vi "Set Cluster Id.vi"(8 "error in (no error)":errorcluster, 11 "cluster id":string) -> (0 "error out":errorcluster)   [LabVIEW 2021, in "NI Discovery V1 Client.lvlib"]
doc: "Advanced use only. Sets the Cluster Id which causes the next discovery client created to refer to a custom discovery service with the given id. This isolates the services launched through the discovery client to that instance."
uses:
  NI Discovery V1 Client.lvlib
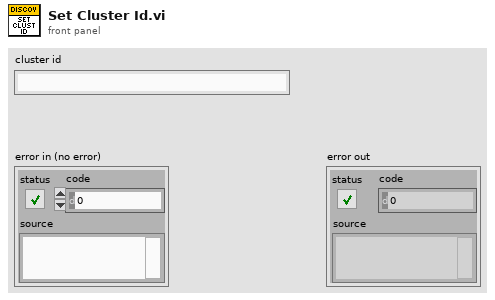
[diagram p1: front panel]
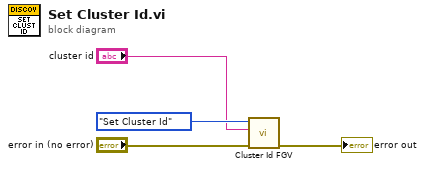
[diagram p0: block diagram]
diagram:
  n1 = call "Cluster Id FGV.vi"("error in (no error)"="error in (no error)", "cluster id"="cluster id", "action"=enum16{"Get Cluster Id", "Set Cluster Id"}."Set Cluster Id") -> ("error out"=→"error out":errorcluster)  [unwired: 7 in, 1 out]
